vi "FlatToRichmeasurement_DataResponse.vi"(5 "OutputClusterType":T1, 11 "InputCluster":T2) -> (3 "OutputCluster":T1)   [LabVIEW 2021, in "Measurement_server.lvlib"]
uses:
  Measurement_server.lvlib
  measurement_DataResponse_Flat.ctl
  measurement_DataResponse.ctl
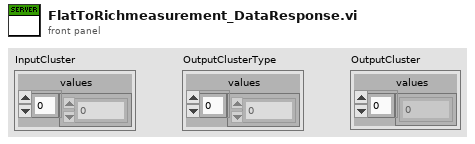
[diagram p1: front panel]
types:
  T1 = typedef "Measurement_server.lvlib/measurement_DataResponse.ctl" = cluster{"values":dbl[]}
  T2 = typedef "Measurement_server.lvlib/measurement_DataResponse_Flat.ctl" = cluster{"values":dbl[]}
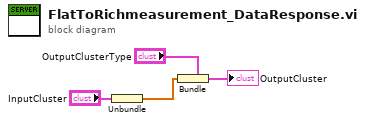
[diagram p0: block diagram]
diagram:
  n1 = Unbundle "Unbundle"("InputCluster") -> ("values"=w1:dbl[])
  n2 = Bundle "Bundle"(cluster="OutputClusterType", "values"=w1) -> (→"OutputCluster":T1)
